vi "MonitorAutoSetting.vi"(8 "error in (no error)":errorcluster) -> (0 "error out":errorcluster)   [LabVIEW 2018]
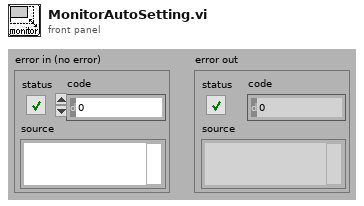
[diagram p1: front panel]
types:
  T1 = typedef "LVPointTypeDef.ctl" = cluster{"Horizontal":i16, "Vertical":i16}
  T2 = typedef "LVRectTypeDef.ctl" = cluster{"Left":i16, "Top":i16, "Right":i16, "Bottom":i16}
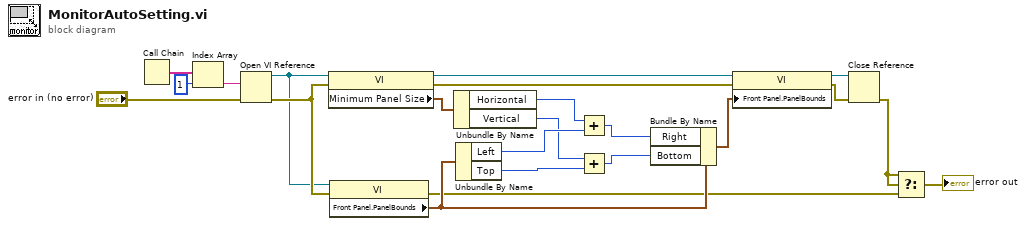
[diagram p0: block diagram]
diagram:
  n1 = Call Chain() -> (call chain=w22:string[])
  n2 = Index Array(array=w22, index=1 ("索引")) -> (element=w20:string)
  n3 = Open VI Reference(vi path=w20, error in (no error)="error in (no error)") -> (vi reference=w3:refnum<vi>, error out=w4:errorcluster)  [unwired: 4 out]
  n4 = property class="VI"(reference=w3, error in=w4) -> (reference out=w11:refnum<vi>, error out=w10:errorcluster, "Minimum Panel Size"=w19:T1)
  n5 = property class="VI"(reference=w3, error in=w4) -> (error out=w7:errorcluster, "Front Panel.PanelBounds"=w14:T2)  [unwired: 1 out]
  n6 = Unbundle By Name(w19) -> ("Horizontal"=w18:i16, "Vertical"=w16:i16)
  n7 = Unbundle By Name(w14) -> ("Left"=w17:i16, "Top"=w15:i16)
  n8 = Add(x=w18, y=w17) -> (x+y=w13:i16)
  n9 = Add(x=w16, y=w15) -> (x+y=w12:i16)
  n10 = Bundle By Name(cluster=w14, "Right"=w13, "Bottom"=w12) -> (w9:T2)
  n11 = property class="VI"(reference=w11, error in=w10, "Front Panel.PanelBounds"=w9) -> (reference out=w8:refnum<vi>, error out=w6:errorcluster)
  n12 = Close Reference(reference=w8, error in (no error)=w6) -> (error out=w5:errorcluster)
  n13 = Select(t=w5, s=w5, f=w7) -> (s? t:f=→"error out":errorcluster)
